vi "Trim String Array.vi"(7 "String Array":string[](array[string])) -> (8 "String Array Trimmed":string[](array[string]))   [LabVIEW 2013]
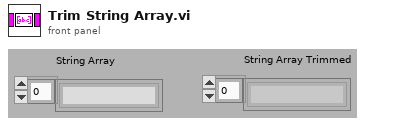
[diagram p1: front panel]
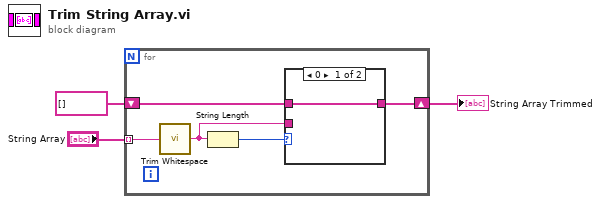
[diagram p0: block diagram]
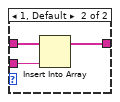
[diagram p2: hidden frame]
diagram:
  n1 = for {
    tunnel: "String Array" -> [w8] mode=indexing
    shift-right: [w6] -> w2
    shift-left: string[] [] ("String Array") -> [w7]
    n2 = call <vilib>:"Trim Whitespace.vi"("string"=w8) -> ("trimmed string"=w4:string)  [unwired: 1 in]
    n3 = String Length(string=w4) -> (length=w5:i32)
    n4 = case shown="0" w5 {
      tunnel: w7 -> [w9 w12]
      tunnel: [w9 w11] -> w6
      tunnel: w4 -> [_ w10]
      frame 0 {
      }
      frame 1, Default {
        n5 = Insert Into Array(array=w12, new element=w10) -> (w11:string[])  [unwired: 1 in]
      }
    }
  }
  "String Array Trimmed" <- w2
